vi "Read DATA_Notifiers.vi"(8 "error in (no error)":errorcluster, 11 "Notifiers in":refnum<class "Notifiers.lvclass">) -> (0 "error out":errorcluster, 2 "DATA":T1, 3 "Notifiers out":refnum<class "Notifiers.lvclass">)   [LabVIEW 2020, in "Data Communication Transmitter.lvlib" / "Notifiers.lvclass"]
doc: "Data cluster accessors to read the data."
uses:
  Classes/Children/Intra-Application/Children/With Data/Children/Notifiers/Notifiers.lvclass
  Classes/Children/Intra-Application/Children/With Data/Children/Notifiers/Notifiers.lvclass/Notifiers.ctl
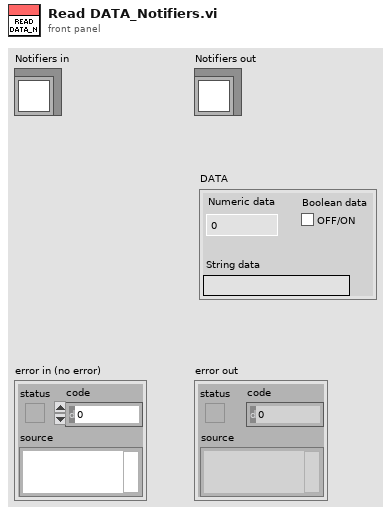
[diagram p1: front panel]
types:
  T1 = cluster{"Numeric data":dbl, "String data":string, "Boolean data":bool}
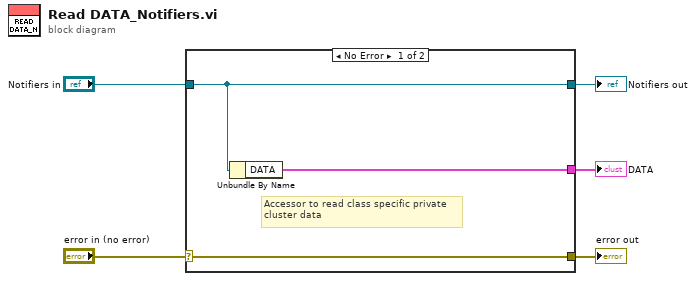
[diagram p0: block diagram]
diagram:
  n1 = case shown="No Error" "error in (no error)" {
    selector: "error in (no error)" -> [w8 w9]
    tunnel: [w8 w9] -> w4
    tunnel: [w7 w10] -> w2
    tunnel: "Notifiers in" -> [w7 w10]
    tunnel: [w6 _] -> w1
    frame No Error {
      # "Accessor to read class specific private\ncluster data"
      n2 = Unbundle By Name(w7) -> ("DATA"=w6:T1)
    }
    frame Error {
    }
  }
  "error out" <- w4
  "Notifiers out" <- w2
  "DATA" <- w1
